vi "IRF(X)PSED Fourier Coefficients.vi"(8 "Error In":errorcluster, 11 "IRF*PSED fixed Parameters":T1={"order"=0, "T"=0.0, "Time Constant Array"=[], "{S_k, C_k, phi_k, e_k} arrays"={"S_k Array"=[], "C_k Array"=[], "phi_k Array"=[], "e_k Array"=[]}, "IRF Extraction Options"={"Time Constant for IRF Extraction"=1e-18, "IRF Order"=0, "Fourier Series Smoothing"=enum."None", "Noise Threshold"=0.0, "Smoothing Width"=0.0, "Fourier Series Truncation"=enum."Automatic", "Truncation Order"=0, "Save Power Spectrum"=FALSE}} {"IRF Extraction Options"."Time Constant for IRF Extraction" format="%#_5g"}) -> (0 "Error Out":errorcluster, 1 "Optimal Order":i32, 2 "[b_k]":dbl[](array[numeric]), 3 "[a_k]":dbl[](array[numeric]), 4 "[s_k]":dbl[](array[numeric]), 6 "Smoothed [s_k]":dbl[](array[numeric]))   [LabVIEW 2019]
uses:
  IRF(X)PSED Fixed Parameters v3.ctl
  IRF(X)PSED Extraction Options.ctl
  Fourier Series Smoothing Option.ctl
  Fourier Series Truncation.ctl
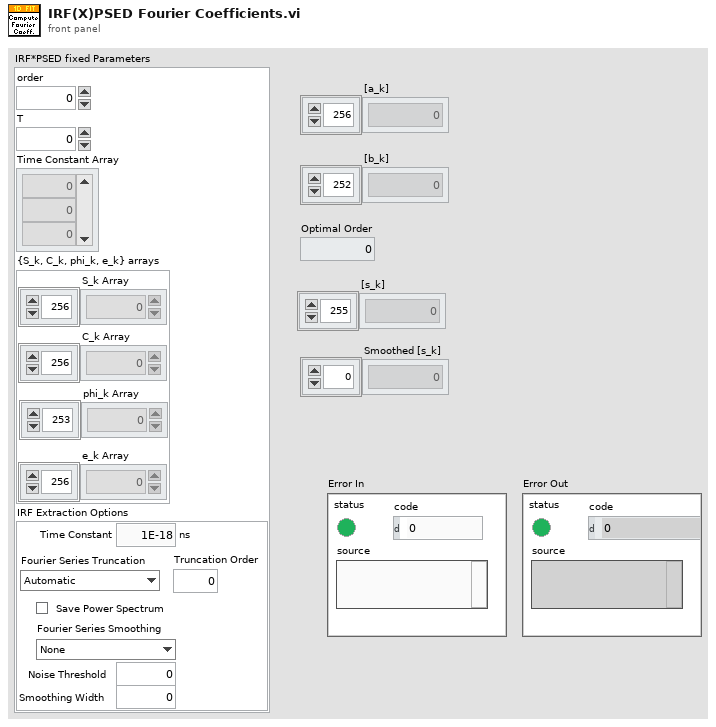
[diagram p1: front panel]
types:
  T1 = typedef "IRF(X)PSED Fixed Parameters v3.ctl" = cluster{"order":i32, "T":dbl, "Time Constant Array":dbl[], "{S_k, C_k, phi_k, e_k} arrays":cluster{"S_k Array":dbl[], "C_k Array":dbl[], "phi_k Array":dbl[], "e_k Array":dbl[]}, "IRF Extraction Options":T2}
  T2 = typedef "IRF(X)PSED Extraction Options.ctl" = cluster{"Time Constant for IRF Extraction":dbl[unit], "IRF Order":i32, "Fourier Series Smoothing":T3, "Noise Threshold":dbl, "Smoothing Width":dbl, "Fourier Series Truncation":T4, "Truncation Order":i32, "Save Power Spectrum":bool}
  T3 = typedef "Fourier Series Smoothing Option.ctl" = enum16{"None", "Lanczos Factors", "Fejer Summation"}
  T4 = typedef "Fourier Series Truncation.ctl" = enum16{"Automatic", "Fixed"}
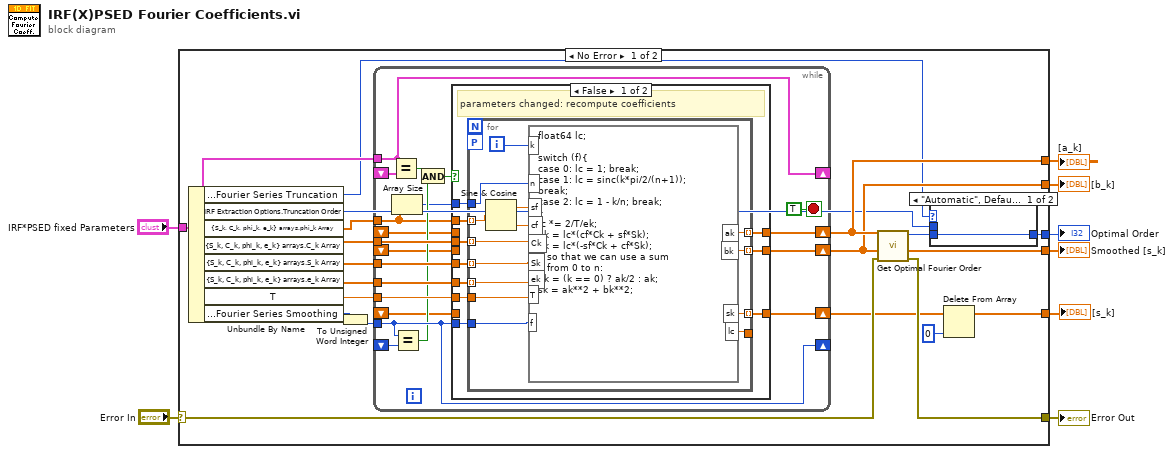
[diagram p0: block diagram]
diagram:
  n1 = case shown="No Error" "Error In" {
    selector: "Error In" -> [w22 w78]
    tunnel: "IRF*PSED fixed Parameters" -> [w28 _]
    tunnel: [w21 w78] -> w6
    tunnel: [w20 _] -> w5
    tunnel: [w16 _] -> w4
    tunnel: [w13 _] -> w3
    tunnel: [w11 _] -> w2
    tunnel: [w17 _] -> w1
    frame No Error {
      n2 = Unbundle By Name(w28) -> ("IRF Extraction Options.Fourier Series Truncation"=w15:T4, "IRF Extraction Options.Truncation Order"=w12:i32, "{S_k, C_k, phi_k, e_k} arrays.phi_k Array"=w26:dbl[], "{S_k, C_k, phi_k, e_k} arrays.C_k Array"=w23:dbl[], "{S_k, C_k, phi_k, e_k} arrays.S_k Array"=w24:dbl[], "{S_k, C_k, phi_k, e_k} arrays.e_k Array"=w25:dbl[], "T"=w27:dbl, "IRF Extraction Options.Fourier Series Smoothing"=w19:T3)
      n3 = To Unsigned Word Integer(number=w19) -> (unsigned 16bit integer=w9:u16)
      n4 = while {
        tunnel: w23 -> [w50]
        tunnel: w24 -> [w49]
        tunnel: w25 -> [w48]
        tunnel: w26 -> [w33]
        tunnel: w27 -> [w45]
        tunnel: w9 -> [w40]
        tunnel: w28 -> [w43]
        shift-right: [w47] -> w20
        shift-left: _ -> [w36]
        shift-right: [w46] -> w16
        shift-left: _ -> [w35]
        shift-right: [w43] -> _
        shift-left: _ -> [w42]
        shift-right: [w40] -> _
        shift-left: _ -> [w41]
        shift-right: [w31] -> w18
        shift-left: _ -> [w34]
        stop <- TRUE stop-if-true
        n5 = Equal?(x=w43, y=w42) -> (x = y?=w39:bool)
        n6 = Array Size(array=w33) -> (size(s)=w32:i32)
        n7 = Equal?(x=w40, y=w41) -> (x = y?=w38:bool)
        n8 = And(x=w39, y=w38) -> (x .and. y?=w37:bool)
        n9 = case shown="False" w37 {
          tunnel: w50 -> [w60 _]
          tunnel: w49 -> [w59 _]
          tunnel: w48 -> [w58 _]
          tunnel: w33 -> [w57 _]
          tunnel: [w53 w77] -> w47
          tunnel: [w54 w76] -> w46
          tunnel: w45 -> [w55 _]
          tunnel: w40 -> [w56 _]
          tunnel: w36 -> [_ w77]
          tunnel: w35 -> [_ w76]
          tunnel: [w52 w75] -> w31
          tunnel: w34 -> [_ w75]
          tunnel: w32 -> [w51 _]
          frame False {
            # "parameters changed: recompute coefficients"
            n10 = for {
              tunnel: w57 -> [w65] mode=indexing
              tunnel: w60 -> [w72] mode=indexing
              tunnel: w59 -> [w71] mode=indexing
              tunnel: [w70] -> w53 mode=indexing
              tunnel: [w69] -> w54 mode=indexing
              tunnel: w56 -> [w67]
              tunnel: w58 -> [w66] mode=indexing
              tunnel: w55 -> [w64]
              tunnel: [w63] -> w52 mode=indexing
              tunnel: w51 -> [w62]
              tunnel: [w61] -> _
              workers-P: _ -> [_]
              i -> [w68]
              n11 = Sine & Cosine(0:w65) -> (1:w74:dbl, 2:w73:dbl)
              n12 = formula code="float64 lc;\n\nswitch (f){\ncase 0: lc = 1; break; \ncase 1: lc = sinc(k*pi/2/(n+1));\nbreak;\ncase 2: lc = 1 - k/n; break;\n}\nlc *= 2/T/ek;\nak = lc*(cf*Ck + sf*Sk);\nbk = lc*(-sf*Ck + cf*Sk);\n// so that we can use a sum\n// from 0 to n:\nak = (k == 0) ? ak/2 : ak;\nsk = ak**2 + bk**2;"("sf"=w74, "cf"=w73, "Ck"=w72, "Sk"=w71, "k"=w68, "f"=w67, "ek"=w66, "T"=w64, "n"=w62) -> ("ak"=w70:dbl, "bk"=w69:dbl, "sk"=w63:dbl, "lc"=w61:dbl)
            }
          }
          frame True {
            # "no need to recompute coefficients"
          }
        }
      }
      n13 = call "Get Optimal Fourier Order.vi"("Error In"=w22, "[b_k]"=w16, "[a_k]"=w20) -> ("Error Out"=w21:errorcluster, "Smoothed Power Spectrum"=w17:dbl[], "Optimal Fourier Order"=w14:i32)  [unwired: 6 in]
      n14 = case shown="\"Automatic\", Default" w15 {
        tunnel: w14 -> [w29 _]
        tunnel: [w29 w30] -> w13
        tunnel: w12 -> [_ w30]
        frame "Automatic", Default {
        }
        frame "Fixed" {
        }
      }
      n15 = Delete From Array(array=w18, index=0) -> (array with subset deleted=w11:dbl[])  [unwired: 1 in, 1 out]
    }
    frame Error {
    }
  }
  "Optimal Order" <- w3
  "Error Out" <- w6
  "[a_k]" <- w5
  "[b_k]" <- w4
  "[s_k]" <- w2
  "Smoothed [s_k]" <- w1
